vi "objectCount.vi"() -> ()   [LabVIEW 2021]
panel:
  out "Count":i16
  out "x = y?":bool[](array[boolean])
  in  "Enter the character/String":string
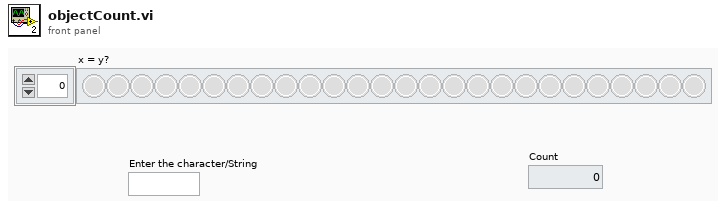
[diagram p1: front panel]
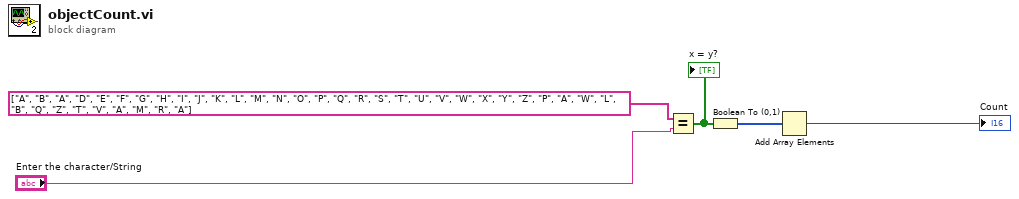
[diagram p0: block diagram]
diagram:
  n1 = Equal?(x=string[] ["A", "B", "A", "D", "E", "F", "G", "H", "I", "J", "K", "L", "M", "N", "O", "P", "Q", "R", "S", "T", "U", "V", "W", "X", "Y", "Z", "P", "A", "W", "L", "B", "Q", "Z", "T", "V", "A", "M", "R", "A"], y="Enter the character/String") -> (x = y?=w3:bool[])
  "x = y?" <- w3
  n2 = Boolean To (0,1)(Boolean=w3) -> (0, 1=w2:i16[])
  n3 = Add Array Elements(numeric array=w2) -> (sum=→"Count":i16)
